vi "Read Msg Output.vi"(11 "Start Msg Output in":refnum<class "Start Msg Output.lvclass">) -> ()   [LabVIEW 2020, in "jettl.lvlib" / "Start jettl Msg.lvlib" / "Start Msg Output.lvlib" / "Start Msg Output.lvclass"]
doc: "jettl 6.14.1.98\nNathan Davis - Nathan Davis\nCopyright (c) 2026, Nathan Davis\nMIT"
uses:
  Start Msg Output.lvclass
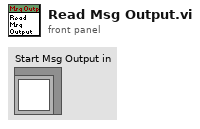
[diagram p1: front panel]
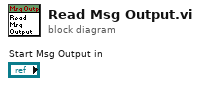
[diagram p0: block diagram]
diagram:
